vi "ctx get expected sync delta.vi"(10 "dest_expected_sync_delta":u16, 11 "context":u32) -> (1 "function return":i32, 2 "dest_expected_sync_delta out":u16, 3 "context out":u32)   [LabVIEW 2019, in "apdm.lvlib"]
doc: "APDM_EXPORT int apdm_ctx_get_expected_sync_delta(apdm_ctx_t context, uint16_t *dest_expected_sync_delta);"
uses:
  apdm.lvlib
  Lee Lab/CP FES Walking 2018/Code/Working/LabVIEW/apdm.dll
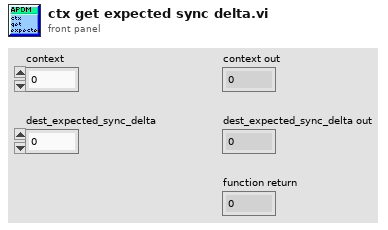
[diagram p1: front panel]
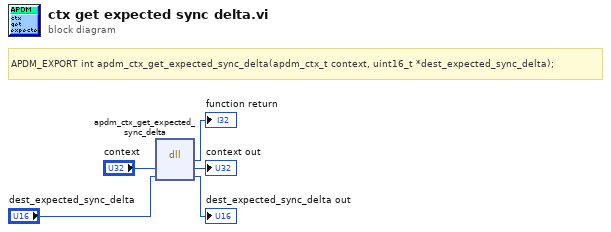
[diagram p0: block diagram]
diagram:
  # "APDM_EXPORT int apdm_ctx_get_expected_sync_delta(apdm_ctx_t context, uint16_t *dest_expected_sync_delta);"
  n1 = dll-call lib="C:/Users/jfalesi/Dropbox/Lee Lab/CP FES Walking 2018/Code/Working/LabVIEW/apdm.*" fn="apdm_ctx_get_expected_sync_delta"("context"="context", "dest_expected_sync_delta"="dest_expected_sync_delta") -> (→"function return":i32, "context"=→"context out":u32, "dest_expected_sync_delta"=→"dest_expected_sync_delta out":u16)  [unwired: 3 in, 2 out]
